vi "Update Chart Display--SubVI.vi"(9 "Length":i32, 10 "Start Index":i32, 11 "Chart Data Array":dbl[][](array[numeric])) -> (3 "Chart Data":dbl[][](array[numeric]))   [LabVIEW 2025, in "Chart.lvlib"]
doc: "<b>Note:</b> This VI was modified by the <b>Validate DQMH Module</b> tool to turn off automatic error handling."
uses:
  Chart.lvlib
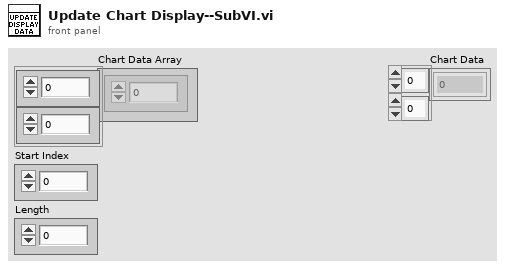
[diagram p1: front panel]
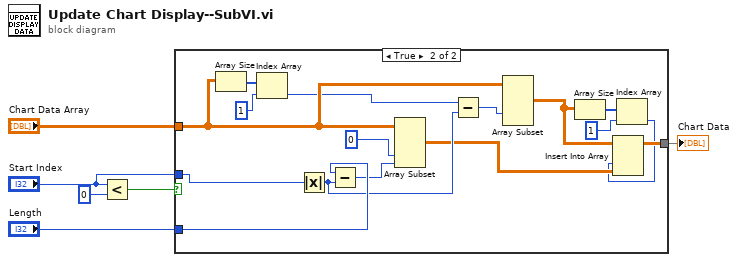
[diagram p0: block diagram]
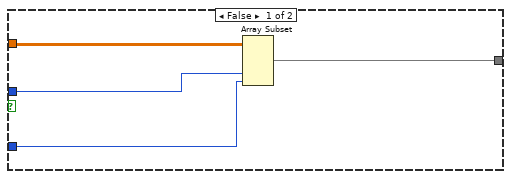
[diagram p2: hidden frame]
diagram:
  n1 = Less?(x="Start Index", y=0) -> (x < y?=w5:bool)
  n2 = case shown="True" w5 {
    tunnel: "Chart Data Array" -> [w10 w12]
    tunnel: "Length" -> [w8 w26]
    tunnel: "Start Index" -> [w7 w25]
    tunnel: [w9 w22] -> w1
    frame False {
      n3 = Array Subset(array=w10, index (col)=w7, length (col)=w8) -> (w9:dbl[][])  [unwired: 2 in]
    }
    frame True {
      n4 = Array Size(array=w12) -> (size(s)=w13:i32[])
      n5 = Index Array(array=w13, index=1) -> (element=w11:i32)
      n6 = Absolute Value(x=w25) -> (abs(x)=w24:i32)
      n7 = Subtract(x=w26, y=w24) -> (x-y=w21:i32)
      n8 = Array Subset(array=w12, index (col)=0 ("index"), length (col)=w21) -> (w23:dbl[][])  [unwired: 2 in]
      n9 = Subtract(x=w11, y=w24) -> (x-y=w19:i32)
      n10 = Array Subset(array=w12, index (col)=w19) -> (w18:dbl[][])  [unwired: 3 in]
      n11 = Array Size(array=w18) -> (size(s)=w17:i32[])
      n12 = Index Array(array=w17, index=1 ("y")) -> (element=w15:i32)
      n13 = Insert Into Array(array=w18, index (col)=w15, new element=w23) -> (w22:dbl[][])  [unwired: 1 in]
    }
  }
  "Chart Data" <- w1
